vi "Match mutiple Pattern.vi"(7 "delimiter (|)":string="|", 8 "offset (0)":i32, 10 "regular expression":string, 11 "string":string) -> (0 "Found?":bool, 1 "after substring":string, 2 "match substring":string, 3 "before substring":string)   [LabVIEW 2017]
uses:
  <userlib>/_OpenG.lib/string/string.llb/Trim Whitespace (String Array)__ogtk.vi
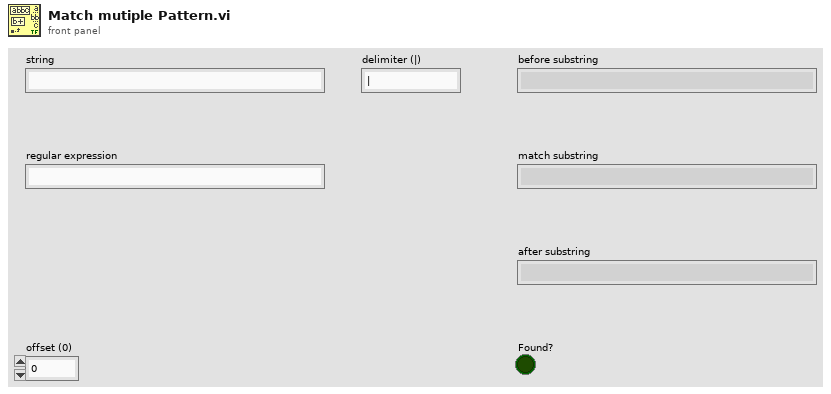
[diagram p1: front panel]
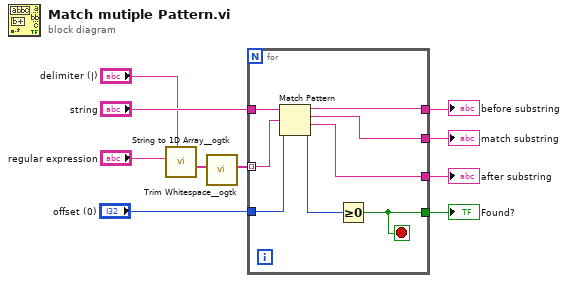
[diagram p0: block diagram]
diagram:
  n1 = call <userlib>:"String to 1D Array__ogtk.vi"("delimiter (Tab)"="delimiter (|)", "string"="regular expression") -> ("Array of Strings"=w2:string[])  [unwired: 9 in]
  n2 = call-poly <userlib>:"Trim Whitespace__ogtk.vi"("String in"=w2) -> ("String out"=w1:string[])  [unwired: 6 in]
  n3 = for {
    tunnel: "offset (0)" -> [w17]
    tunnel: [w14] -> w6
    tunnel: [w11] -> w5
    tunnel: "string" -> [w18]
    tunnel: [w16] -> w8
    tunnel: w1 -> [w12] mode=indexing
    tunnel: [w15] -> w7
    stop <- w11 stop-if-true
    n4 = Match Pattern(string=w18, regular expression=w12, offset (0)=w17) -> (before substring=w16:string, match substring=w15:string, after substring=w14:string, offset past match=w13:i32)
    n5 = Greater Or Equal To 0?(x=w13) -> (x >= 0?=w11:bool)
  }
  "before substring" <- w8
  "match substring" <- w7
  "after substring" <- w6
  "Found?" <- w5
